vi "getStatus_action.vi"(0 "HGF_AVT_F033B":refnum<class "HGF_AVT_F033B.lvclass">, 5 "error in (no error)":errorcluster) -> (13 "Lost Counter":T1, 14 "dup HGF_AVT_F033B":refnum<class "HGF_AVT_F033B.lvclass">, 15 "Acquiring?":bool, 16 "Last Valid Buffer Index":u32, 17 "Last Valid Buffer Number":u32, 19 "error out":errorcluster)   [LabVIEW 2014, in "HGF_IMAQ.lvlib" / "HGF_AVT_F033B.lvclass"]
doc: "Returns status information about the acquisition, such as the state of the acquisition and the last valid buffer acquired."
uses:
  HGF_AVT_F033B.lvclass
  <resource>/objmgr/imaqdx.rc
  HGF_ImaqDx/HGF_ImaqDx.lvclass
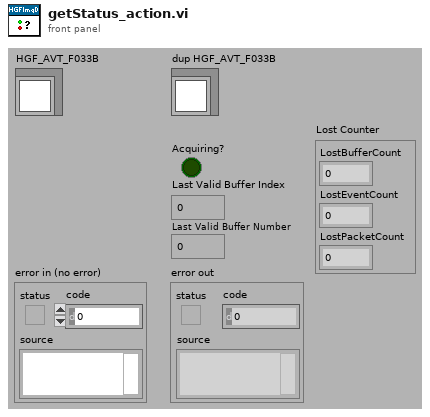
[diagram p1: front panel]
types:
  T1 = cluster{"LostBufferCount":u32, "LostEventCount":u32, "LostPacketCount":u32}
  T2 = typedef "IMAQdx.ctl" = refnum<k21>
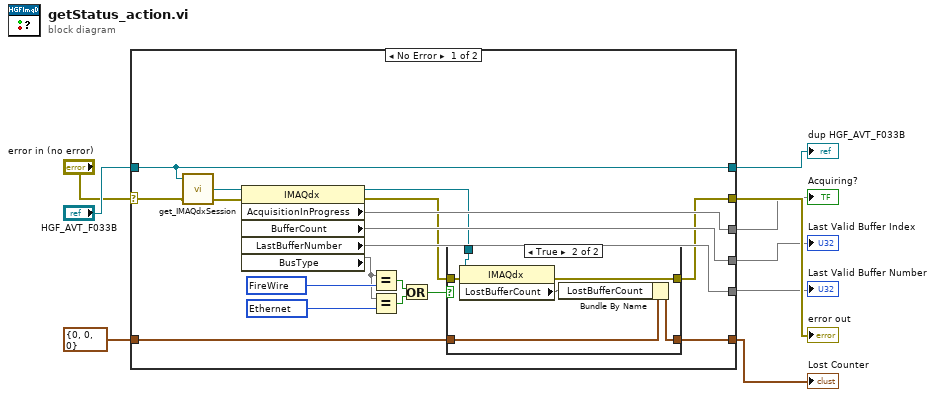
[diagram p0: block diagram]
diagram:
  n1 = case shown="No Error" "error in (no error)" {
    selector: "error in (no error)" -> [w13 w37]
    tunnel: "HGF_AVT_F033B" -> [w10 w38]
    tunnel: [w27 _] -> w1
    tunnel: [w23 _] -> w2
    tunnel: [w24 _] -> w3
    tunnel: [w14 w37] -> w6
    tunnel: [w10 w38] -> w5
    tunnel: [w26 w36] -> w4
    tunnel: T1 {"LostBufferCount"=0, "LostEventCount"=0, "LostPacketCount"=0} ("Lost") -> [w25 w36]
    frame No Error {
      w20 = u32 825440564 items=["FireWire"=825440564, "Ethernet"=1768977972] ("BusType")
      w18 = u32 1768977972 items=["FireWire"=825440564, "Ethernet"=1768977972] ("BusType")
      n2 = call "get_IMAQdxSession.vi"("error in (no error)"=w13, "HGF_ImaqDx in"=w10) -> ("error out"=w12:errorcluster, "IMAQdx Session"=w11:T2)  [unwired: 1 in, 1 out]
      n3 = property class="IMAQdx"(reference=w11, error in=w12) -> (reference out=w22:T2, error out=w21:errorcluster, "AcquisitionInProgress"=w27, "BufferCount"=w23, "LastBufferNumber"=w24, "BusType"=w19)
      n4 = Equal?(x=w19, y=w20) -> (x = y?=w17:bool)
      n5 = Equal?(x=w19, y=w18) -> (x = y?=w16:bool)
      n6 = Or(x=w17, y=w16) -> (x .or. y?=w15:bool)
      n7 = case shown="True" w15 {
        tunnel: [w29 w35] -> w26
        tunnel: w25 -> [w29 w34]
        tunnel: w22 -> [_ w33]
        tunnel: w21 -> [w28 w31]
        tunnel: [w28 w30] -> w14
        frame False {
        }
        frame True {
          n8 = property class="IMAQdx"(reference=w33, error in=w31) -> (error out=w30:errorcluster, "LostBufferCount"=w32)  [unwired: 1 out]
          n9 = Bundle By Name(cluster=w34, "LostBufferCount"=w32) -> (w35:T1)
        }
      }
    }
    frame Error {
    }
  }
  "error out" <- w6
  "dup HGF_AVT_F033B" <- w5
  "Acquiring?" <- w1
  "Last Valid Buffer Index" <- w2
  "Last Valid Buffer Number" <- w3
  "Lost Counter" <- w4
